vi "Set cif_manager_PluginTypeReply.vi"(7 "Complete Call (T)":bool=TRUE, 8 "error in (no error)":errorcluster, 10 "package_templatemessage":T1, 11 "gRPCid":T5) -> (0 "error out":errorcluster)   [LabVIEW 2021, in "CIF_Launcher_server.lvlib"]
uses:
  CIF_Launcher_server.lvlib
  <vilib>/gRPC/LabVIEW gRPC Library/Shared/grpcId.ctl
  cif_manager_PluginTypeReply.ctl
  cif_manager_PluginType.ctl
  cif_common_ShortVersion.ctl
  cif_manager_PluginMetadata.ctl
  cif_manager_PluginTypeReply_Flat.ctl
  cif_manager_PluginType_Flat.ctl
  cif_common_ShortVersion_Flat.ctl
  cif_manager_PluginMetadata_Flat.ctl
  dcc74a39-081a-4bdd-860b-8ed792803c96.vi
  RichToFlatcif_manager_PluginType.vi
  <vilib>/gRPC/LabVIEW gRPC Library/Shared/TranslateGrpcError.vi
  RichToFlatcif_common_ShortVersion.vi
  RichToFlatcif_manager_PluginMetadata.vi
  <vilib>/gRPC/LabVIEW gRPC Library/Server API/Server/Get Server DLL Path.vi
  <vilib>/Utility/error.llb/Error Cluster From Error Code.vi
  <vilib>/gRPC/LabVIEW gRPC Library/grpc-lvsupport-release.lvlib
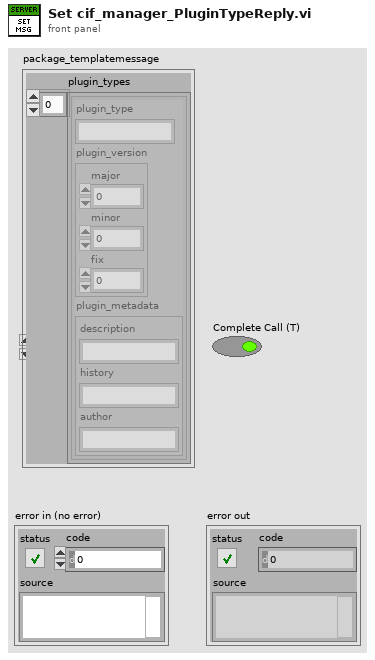
[diagram p1: front panel]
types:
  T1 = typedef "CIF_Launcher_server.lvlib/cif_manager_PluginTypeReply.ctl" = cluster{"plugin_types":T2[]}
  T2 = typedef "CIF_Launcher_server.lvlib/cif_manager_PluginType.ctl" = cluster{"plugin_type":string, "plugin_version":T3, "plugin_metadata":T4}
  T3 = typedef "CIF_Launcher_server.lvlib/cif_common_ShortVersion.ctl" = cluster{"major":u32, "minor":u32, "fix":u32}
  T4 = typedef "CIF_Launcher_server.lvlib/cif_manager_PluginMetadata.ctl" = cluster{"description":string, "history":string, "author":string}
  T5 = typedef "grpc-lvsupport-release.lvlib/grpcId.ctl" = u64
  T6 = typedef "CIF_Launcher_server.lvlib/cif_manager_PluginTypeReply_Flat.ctl" = cluster{"plugin_types":T7[]}
  T7 = typedef "CIF_Launcher_server.lvlib/cif_manager_PluginType_Flat.ctl" = cluster{"plugin_type":string, "plugin_version":T8, "plugin_metadata":T9}
  T8 = typedef "CIF_Launcher_server.lvlib/cif_common_ShortVersion_Flat.ctl" = cluster{"major":u32, "minor":u32, "fix":u32}
  T9 = typedef "CIF_Launcher_server.lvlib/cif_manager_PluginMetadata_Flat.ctl" = cluster{"description":string, "history":string, "author":string}
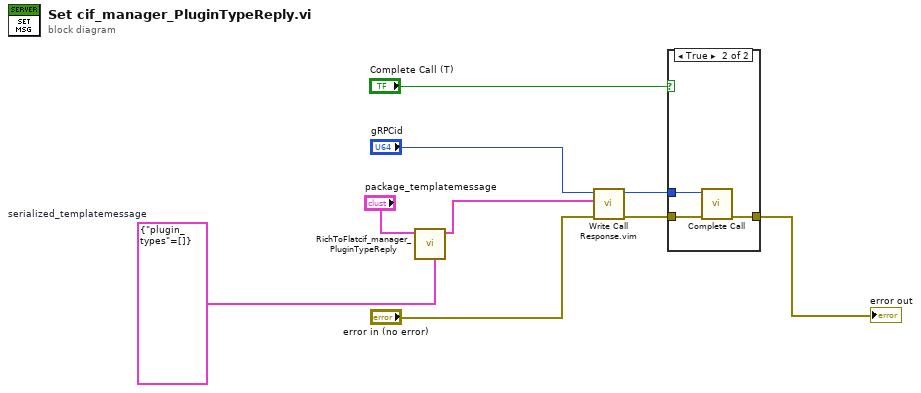
[diagram p0: block diagram]
diagram:
  w2 = T6 {"plugin_types"=[]}  # serialized_templatemessage
  n1 = call "RichToFlatcif_manager_PluginTypeReply.vi"("OutputClusterType"=w2, "InputCluster"="package_templatemessage") -> ("OutputCluster"=w1:T6)  [unwired: 9 in]
  n2 = call "Write Call Response.vim"("error in"="error in (no error)", "Response Data"=w1, "gRPCid in"="gRPCid") -> ("error out"=w6:errorcluster, "gRPCid out"=w7:T5)  [unwired: 7 in]
  n3 = case shown="True" "Complete Call (T)" {
    tunnel: [w10 w13] -> w9
    tunnel: w7 -> [_ w12]
    tunnel: w6 -> [w10 w11]
    frame False {
    }
    frame True {
      n4 = call <vilib>:"Complete Call.vi"("gRPCid"=w12, "error in"=w11) -> ("error out"=w13:errorcluster)  [unwired: 8 in]
    }
  }
  "error out" <- w9
